vi "TuneTempController_v00.vi"() -> ()   [LabVIEW 2011]
panel:
  in  "Write when event occurs":bool
  in  "OK":bool
  in  "Write":bool
  in  "Read Current Value":bool
  out "Value Array":dbl[](array[numeric])
  out "Transfer Bar":u8(slide) caption="Transfer progress..." scale=0.0..100.0
  in  "New Value":dbl caption="Value:"
  in  "Upload Values":bool
  in  "Download Values":bool
  in  "Load Configuration":bool
  in  "Cancel":bool
  in  "Parameters":i32(listbox)
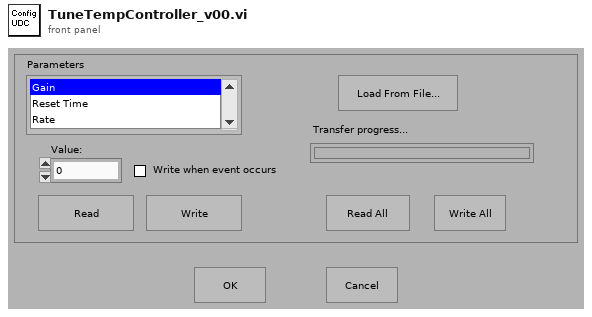
[diagram p1: front panel]
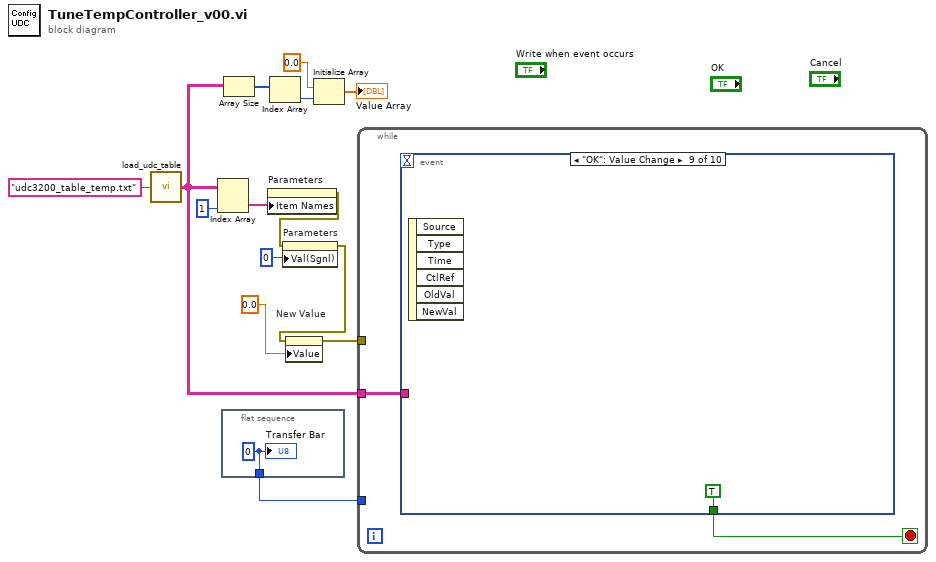
[diagram p0: block diagram]
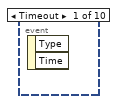
[diagram p2: hidden frame]
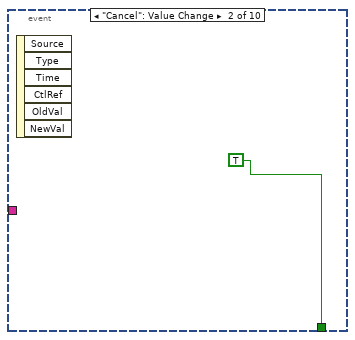
[diagram p3: hidden frame]
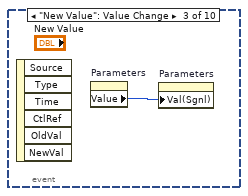
[diagram p4: hidden frame]
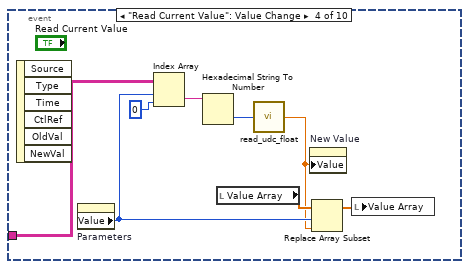
[diagram p5: hidden frame]
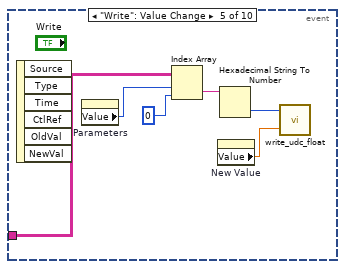
[diagram p6: hidden frame]
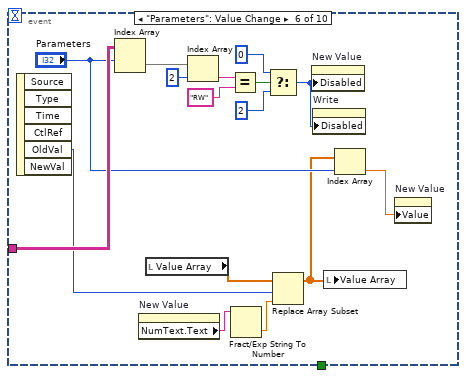
[diagram p7: hidden frame]
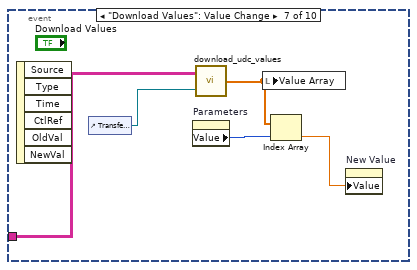
[diagram p8: hidden frame]
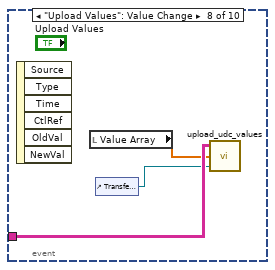
[diagram p9: hidden frame]
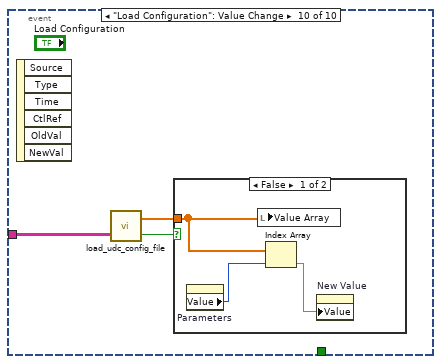
[diagram p10: hidden frame]
diagram:
  n1 = call "load_udc_table.vi"("name or relative path"="udc3200_table_temp.txt") -> ("UDC Table"=w10:string[][])
  n2 = Index Array(array=w10, index (col)=1 ("disabled index (col)")) -> (element=w13:string[])  [unwired: 1 in]
  n3 = flat-sequence {
    tunnel: [w15] -> w4
    frame #0 {
      w15 = u8 0 ("Transfer in progress...")
      "Transfer Bar" <- w15
    }
  }
  n4 = Array Size(array=w10) -> (size(s)=w9:i32[])
  n5 = property on="Parameters" class="LstBox (strict)"("Item Names"=w13) -> (error out=w11:errorcluster)  [unwired: 2 in, 1 out]
  n6 = Index Array(array=w9) -> (element=w8:i32)  [unwired: 1 in]
  n7 = property on="Parameters" class="LstBox (strict)"(error in=w11, "Val(Sgnl)"=0 ("Parameters")) -> (error out=w1:errorcluster)  [unwired: 1 in, 1 out]
  n8 = property on="New Value" class="DigNum (strict)"(error in=w1, "Value"=0.0 ("Current Value")) -> (error out=w5:errorcluster)  [unwired: 1 in, 1 out]
  n9 = Initialize Array(0.0, w8) -> (→"Value Array":dbl[])
  n10 = while {
    tunnel: w10 -> [w17]
    tunnel: w5 -> [_]
    tunnel: w4 -> [_]
    stop <- w16 stop-if-true
    n11 = event shown="[8] \"OK\": Value Change" {
      selector: _ -> [_ _ _ _ _ _ _ _ _ _]
      dyn-events: _ -> [_ _ _ _ _ _ _ _ _ _]
      timeout: _ -> [_ _ _ _ _ _ _ _ _ _]
      tunnel: w17 -> [_ _ _ w27 w33 w49 w54 w57 _ w61]
      tunnel: [_ TRUE ("is done") _ _ _ _ _ _ TRUE ("is done") _] -> w16
      event Timeout {
        n12 = event-data() -> ()  [unwired: 3 out]
      }
      event "Cancel": Value Change {
        n13 = event-data() -> ()  [unwired: 7 out]
      }
      event "New Value": Value Change {
        n14 = event-data() -> ()  [unwired: 7 out]
        n15 = property on="Parameters" class="LstBox (strict)"() -> ("Value"=w19:i32)  [unwired: 2 in, 2 out]
        n16 = property on="Parameters" class="LstBox (strict)"("Val(Sgnl)"=w19) -> ()  [unwired: 2 in, 2 out]
      }
      event "Read Current Value": Value Change {
        n17 = event-data() -> ()  [unwired: 7 out]
        n18 = property on="Parameters" class="LstBox (strict)"() -> ("Value"=w22:i32)  [unwired: 2 in, 2 out]
        n19 = Index Array(array=w27, index (row)=w22, index (col)=0 ("disabled index (col)")) -> (element=w25:string)
        n20 = Hexadecimal String To Number(string=w25) -> (number=w24:u32)  [unwired: 3 out]
        n21 = local read "Value Array"() -> (w23:dbl[])
        n22 = call "read_udc_float.vi"("Hex Address"=w24) -> ("Value"=w21:dbl)
        n23 = property on="New Value" class="DigNum (strict)"("Value"=w21) -> ()  [unwired: 2 in, 2 out]
        n24 = Replace Array Subset(array=w23, new element=w21, index=w22) -> (w20:dbl[])
        n25 = local write "Value Array"(w20) -> ()
      }
      event "Write": Value Change {
        n26 = event-data() -> ()  [unwired: 7 out]
        n27 = property on="Parameters" class="LstBox (strict)"() -> ("Value"=w29:i32)  [unwired: 2 in, 2 out]
        n28 = Index Array(array=w33, index (row)=w29, index (col)=0 ("disabled index (col)")) -> (element=w31:string)
        n29 = property on="New Value" class="DigNum (strict)"() -> ("Value"=w28:dbl)  [unwired: 2 in, 2 out]
        n30 = Hexadecimal String To Number(string=w31) -> (number=w30:u32)  [unwired: 3 out]
        n31 = call "write_udc_float.vi"("Value"=w28, "Hex Address"=w30) -> ()  [unwired: 1 out]
      }
      event "Parameters": Value Change {
        n32 = event-data() -> ("OldVal"=w40:i32)  [unwired: 6 out]
        n33 = Index Array(array=w49, index (row)="Parameters") -> (element=w42:string[])  [unwired: 1 in]
        n34 = property on="New Value" class="DigNum (strict)"() -> ("NumText.Text"=w39:string)  [unwired: 2 in, 2 out]
        n35 = local read "Value Array"() -> (w36:dbl[])
        n36 = Index Array(array=w42, index=2) -> (element=w47:string)
        n37 = Equal?(x=w47, y="RW") -> (x = y?=w45:bool)
        n38 = Fract/Exp String To Number(string=w39) -> (number=w37:dbl)  [unwired: 4 out]
        n39 = Select(t=u8 0 ("Disabled"), s=w45, f=u8 2 ("Disabled")) -> (s? t:f=w34:u8)
        n40 = Replace Array Subset(array=w36, new element=w37, index=w40) -> (w35:dbl[])
        n41 = property on="New Value" class="DigNum (strict)"("Disabled"=w34) -> ()  [unwired: 2 in, 2 out]
        n42 = property on="Write" class="Bool"("Disabled"=w34) -> ()  [unwired: 2 in, 2 out]
        n43 = local write "Value Array"(w35) -> ()
        n44 = Index Array(array=w35, index="Parameters") -> (element=w38:dbl)
        n45 = property on="New Value" class="DigNum (strict)"("Value"=w38) -> ()  [unwired: 2 in, 2 out]
      }
      event "Download Values": Value Change {
        n46 = event-data() -> ()  [unwired: 7 out]
        n47 = control-ref of="Transfer Bar"() -> (w53:refnum<vi>)
        n48 = property on="Parameters" class="LstBox (strict)"() -> ("Value"=w51:i32)  [unwired: 2 in, 2 out]
        n49 = call "download_udc_values.vi"("Transfer Bar"=w53, "UDC Table"=w54) -> ("Value Array"=w52:dbl[])
        n50 = local write "Value Array"(w52) -> ()
        n51 = Index Array(array=w52, index=w51) -> (element=w50:dbl)
        n52 = property on="New Value" class="DigNum (strict)"("Value"=w50) -> ()  [unwired: 2 in, 2 out]
      }
      event "Upload Values": Value Change {
        n53 = event-data() -> ()  [unwired: 7 out]
        n54 = local read "Value Array"() -> (w55:dbl[])
        n55 = control-ref of="Transfer Bar"() -> (w56:refnum<vi>)
        n56 = call "upload_udc_values.vi"("Transfer Bar"=w56, "Value Array"=w55, "UDC Table"=w57) -> ()  [unwired: 1 out]
      }
      event "OK": Value Change {
        n57 = event-data() -> ()  [unwired: 7 out]
      }
      event "Load Configuration": Value Change {
        n58 = event-data() -> ()  [unwired: 7 out]
        n59 = call "load_udc_config_file.vi"("UDC Table"=w61) -> ("Cancelled"=w60:bool, "Array"=w59:dbl[])  [unwired: 1 in]
        n60 = case shown="False" w60 {
          tunnel: w59 -> [w64 _]
          frame False {
            n61 = property on="Parameters" class="LstBox (strict)"() -> ("Value"=w63:i32)  [unwired: 2 in, 2 out]
            n62 = local write "Value Array"(w64) -> ()
            n63 = Index Array(array=w64, index=w63) -> (element=w62:dbl)
            n64 = property on="New Value" class="DigNum (strict)"("Value"=w62) -> ()  [unwired: 2 in, 2 out]
          }
          frame True {
          }
        }
      }
    }
  }
